vi "getRelayCardSlot.vi"(1 "Relay Card Index":i32) -> (0 "Slot":u16)   [LabVIEW 2011]
uses:
  globals.vi
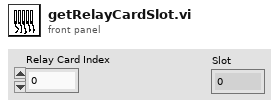
[diagram p1: front panel]
types:
  T1 = cluster{"Relay Card Slots":cluster{"Card 1":u16, "Card 2":u16, "Card 3":u16, "Card 4":u16, "Card 5":u16}, "A/D Card Slots":cluster{"Scanner":u16, "High-Speed A/D":u16, "Timer":u16}, "D/A Cards":cluster{"Quad (10-bit) D/A Card Slots":cluster{"Card 1":u16, "Card 2":u16, "Card 3":u16, "Card 4":u16, "Card 5":u16}, "Single (12-bit) D/A Card Slot":cluster{"Card 6":u16}}}
  T2 = cluster{"Card 1":u16, "Card 2":u16, "Card 3":u16, "Card 4":u16, "Card 5":u16}
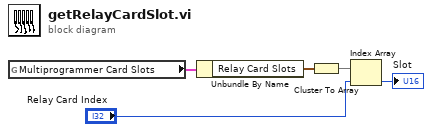
[diagram p0: block diagram]
diagram:
  n1 = global read "globals.vi" "Multiprogrammer Card Slots"() -> (w2:T1)
  n2 = Unbundle By Name(w2) -> ("Relay Card Slots"=w1:T2)
  n3 = Cluster To Array(cluster=w1) -> (array=w3:u16[])
  n4 = Index Array(array=w3, index="Relay Card Index") -> (element=→"Slot":u16)
